vi "Many Nested Cases.vi"() -> ()   [LabVIEW 2024]
panel:
  in  "Numeric Control":dbl
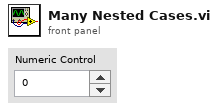
[diagram p1: front panel]
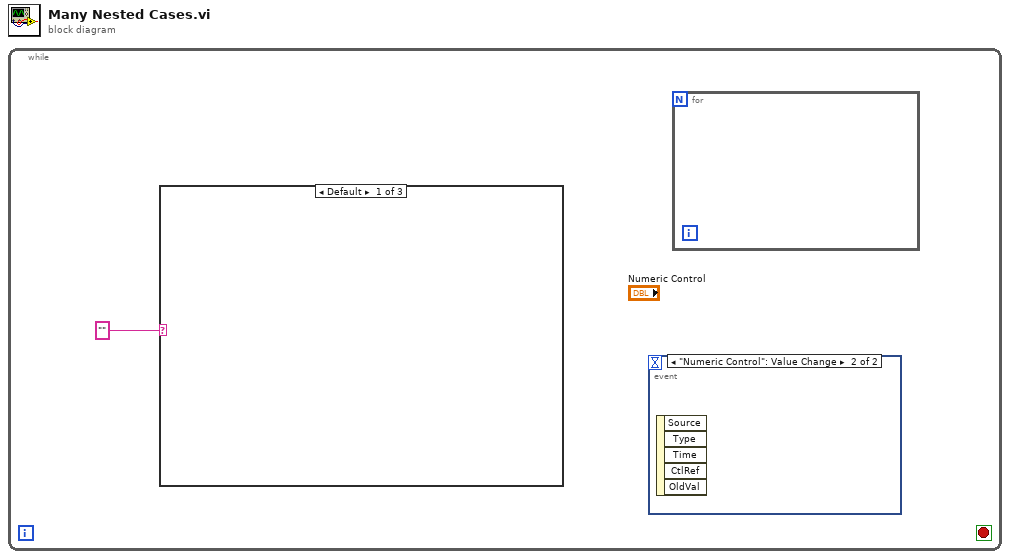
[diagram p0: block diagram]
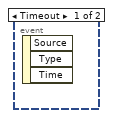
[diagram p2: hidden frame]
diagram:
  n1 = while {
    stop <- _ stop-if-true
    n2 = case shown="Default" "" {
      frame Default {
      }
      frame "False" {
        n3 = case shown="True" {
          selector: _ -> [_ _]
          frame False {
          }
          frame True {
            n4 = case shown="True" {
              selector: _ -> [_ _]
              frame False {
              }
              frame True {
              }
            }
          }
        }
      }
      frame "True" {
      }
    }
    n5 = event shown="[1] \"Numeric Control\": Value Change" {
      selector: _ -> [_ _]
      dyn-events: _ -> [_ _]
      timeout: _ -> [_ _]
      event Timeout {
        n6 = event-data() -> ()  [unwired: 1 in, 3 out]
      }
      event "Numeric Control": Value Change {
        n7 = event-data() -> ()  [unwired: 1 in, 5 out]
      }
    }
    n8 = for {
    }
  }
